vi "get_precision.vi"(8 "error in (no error)":errorcluster caption="entrée d'erreur (pas d'erreur)", 11 "PCA.lvclass 2":refnum<class "PCA.lvclass">) -> (0 "error out":errorcluster caption="sortie d'erreur", 2 "cov":dbl[][](array[numeric]), 3 "PCA.lvclass":refnum<class "PCA.lvclass">)   [LabVIEW 2020, in "PCA.lvclass"]
doc: "Compute data precision matrix with the generative model.\n\n Equals the inverse of the covariance but computed with\n the matrix inversion lemma for efficiency.\n\n Returns\n -------\n precision : array, shape=(n_features, n_features)\n Estimated precision of data."
uses:
  PCA.lvclass
  C:/Users/cipop/TDF Dropbox/2_Technologies de France/1 - Services et Etudes/PLAIY/2 - DEV/PLAIYLAB/code/Python/Python.lvclass
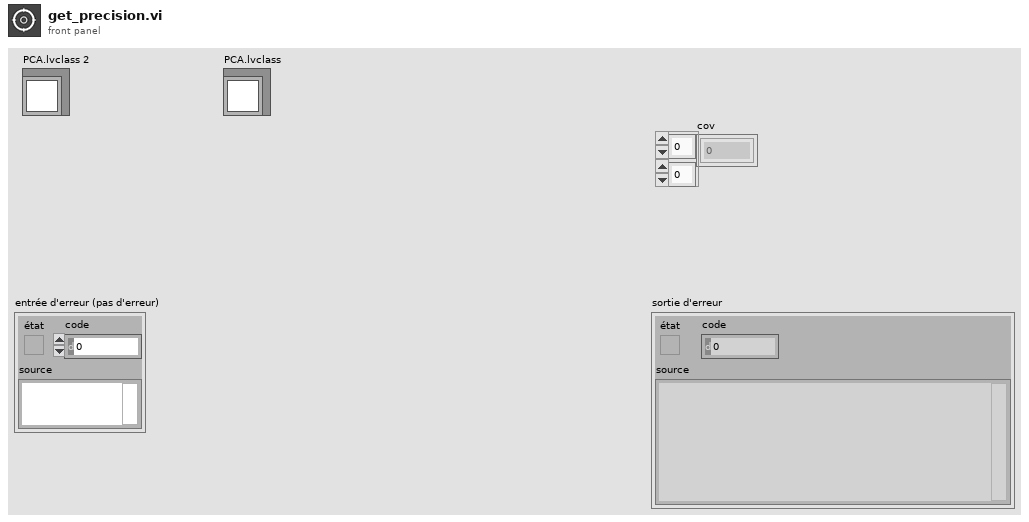
[diagram p1: front panel]
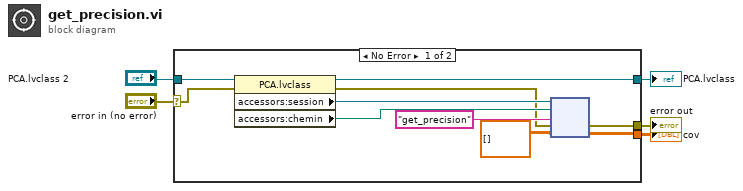
[diagram p0: block diagram]
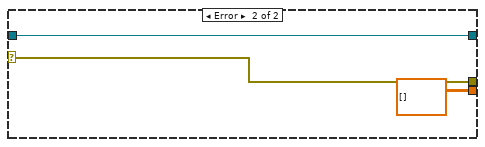
[diagram p2: hidden frame]
diagram:
  n1 = case shown="No Error" "error in (no error)" {
    selector: "error in (no error)" -> [w10 w18]
    tunnel: [w14 w18] -> w4
    tunnel: [w13 w17] -> w1
    tunnel: "PCA.lvclass 2" -> [w8 w17]
    tunnel: [w6 dbl[][] []] -> w3
    frame No Error {
      n2 = property class="PCA.lvclass"(reference=w8, error in=w10) -> (reference out=w13:refnum<class "PCA.lvclass">, error out=w9:errorcluster, "accessors:session"=w12:refnum<k35>, "accessors:chemin"=w11:path)
      n3 = node(w12, w11, "get_precision" ("nom de la fonction"), w9, dbl[][] []) -> (w14:errorcluster, w6:dbl[][])  [unwired: 3 out]
    }
    frame Error {
    }
  }
  "error out" <- w4
  "cov" <- w3
  "PCA.lvclass" <- w1
